vi "Set B.vi"(0 "VISA resource name in":refnum<visa-resource-name>, 7 "Sweep rate":dbl=0.1, 9 "target field":dbl format="%#_13g", 11 "error in":errorcluster) -> (4 "VISA resource name out":refnum<visa-resource-name>, 14 "Response":string, 15 "error out":errorcluster)   [LabVIEW 2021]
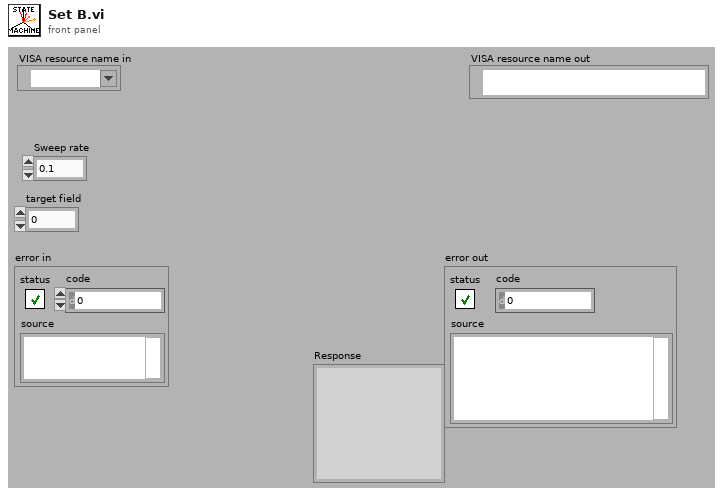
[diagram p1: front panel]
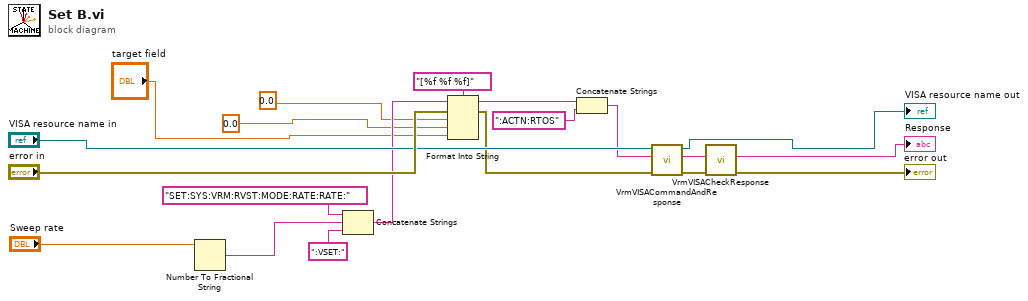
[diagram p0: block diagram]
diagram:
  n1 = Number To Fractional String(number="Sweep rate") -> (F-format string=w5:string)  [unwired: 3 in]
  n2 = Concatenate Strings("SET:SYS:VRM:RVST:MODE:RATE:RATE:", w5, ":VSET:") -> (w4:string)
  n3 = Format Into String(format string="[%f %f %f]", initial string=w4, error in="error in", 0.0, 0.0, "target field") -> (resulting string=w12:string, error out=w13:errorcluster)
  n4 = Concatenate Strings(w12, ":ACTN:RTOS") -> (w14:string)
  n5 = call "VrmVISACommandAndResponse.vi"("error in (no error)"=w13, "Command"=w14, "VISA resource name in"="VISA resource name in") -> ("error out"=w9:errorcluster, "Response"=w8:string, "VISA resource name out"=→"VISA resource name out":refnum<visa-resource-name>)  [unwired: 6 in]
  n6 = call "VrmVISACheckResponse.vi"("error in (no error)"=w9, "Response"=w8) -> ("error out"=→"error out":errorcluster, "Response out"=→"Response":string)  [unwired: 8 in]
